vi "felhasználókl.vi"() -> ()   [LabVIEW 2015]
panel:
  in  "Tab Control":T1(tab)
  out "Array":T2(array[cluster])
  in  "Felhasználó törlése":bool
  in  "Felhasználó módosítása":bool
  in  "Felhasználó hozzáadása":bool
  in  "Felhasználó kiválasztása":string(combo)
  in  "peoples mod":T3
  in  "peoples ins":T3
  in  "Hét kiválasztása":string(combo)
  out "Waveform Chart":waveform(i32)[](graph)
  in  "Felhasználó":string
  out "Mostani hét":string
  out "Array 2":T4(array[cluster]) {"Date" format="%<%H:%M\n%Y/%m/%d>T"; "Time" format="%<%H:%M>T"}
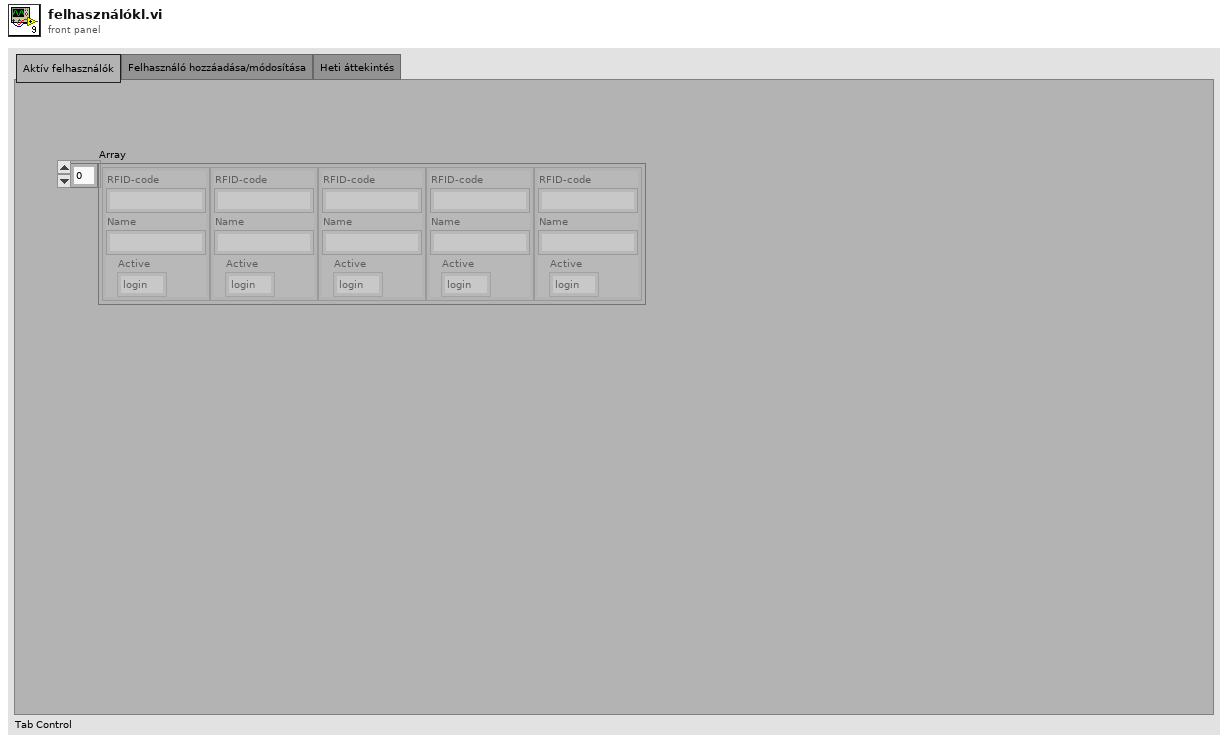
[diagram p1: front panel]
types:
  T1 = enum32{"Aktív felhasználók", "Felhasználó hozzáadása/módosítása", "Heti áttekintés"}
  T2 = cluster{"RFID-code":string, "Name":string, "Active":enum16{"login", "logout"}}[]
  T3 = cluster{"RFID-code":string, "Name":string, "Active":enum16{"login", "logout"}}
  T4 = cluster{"Name":string, "Date":timestamp, "Time":timestamp}[]
  T5 = cluster{"Name":string, "Date":timestamp, "Time":timestamp}
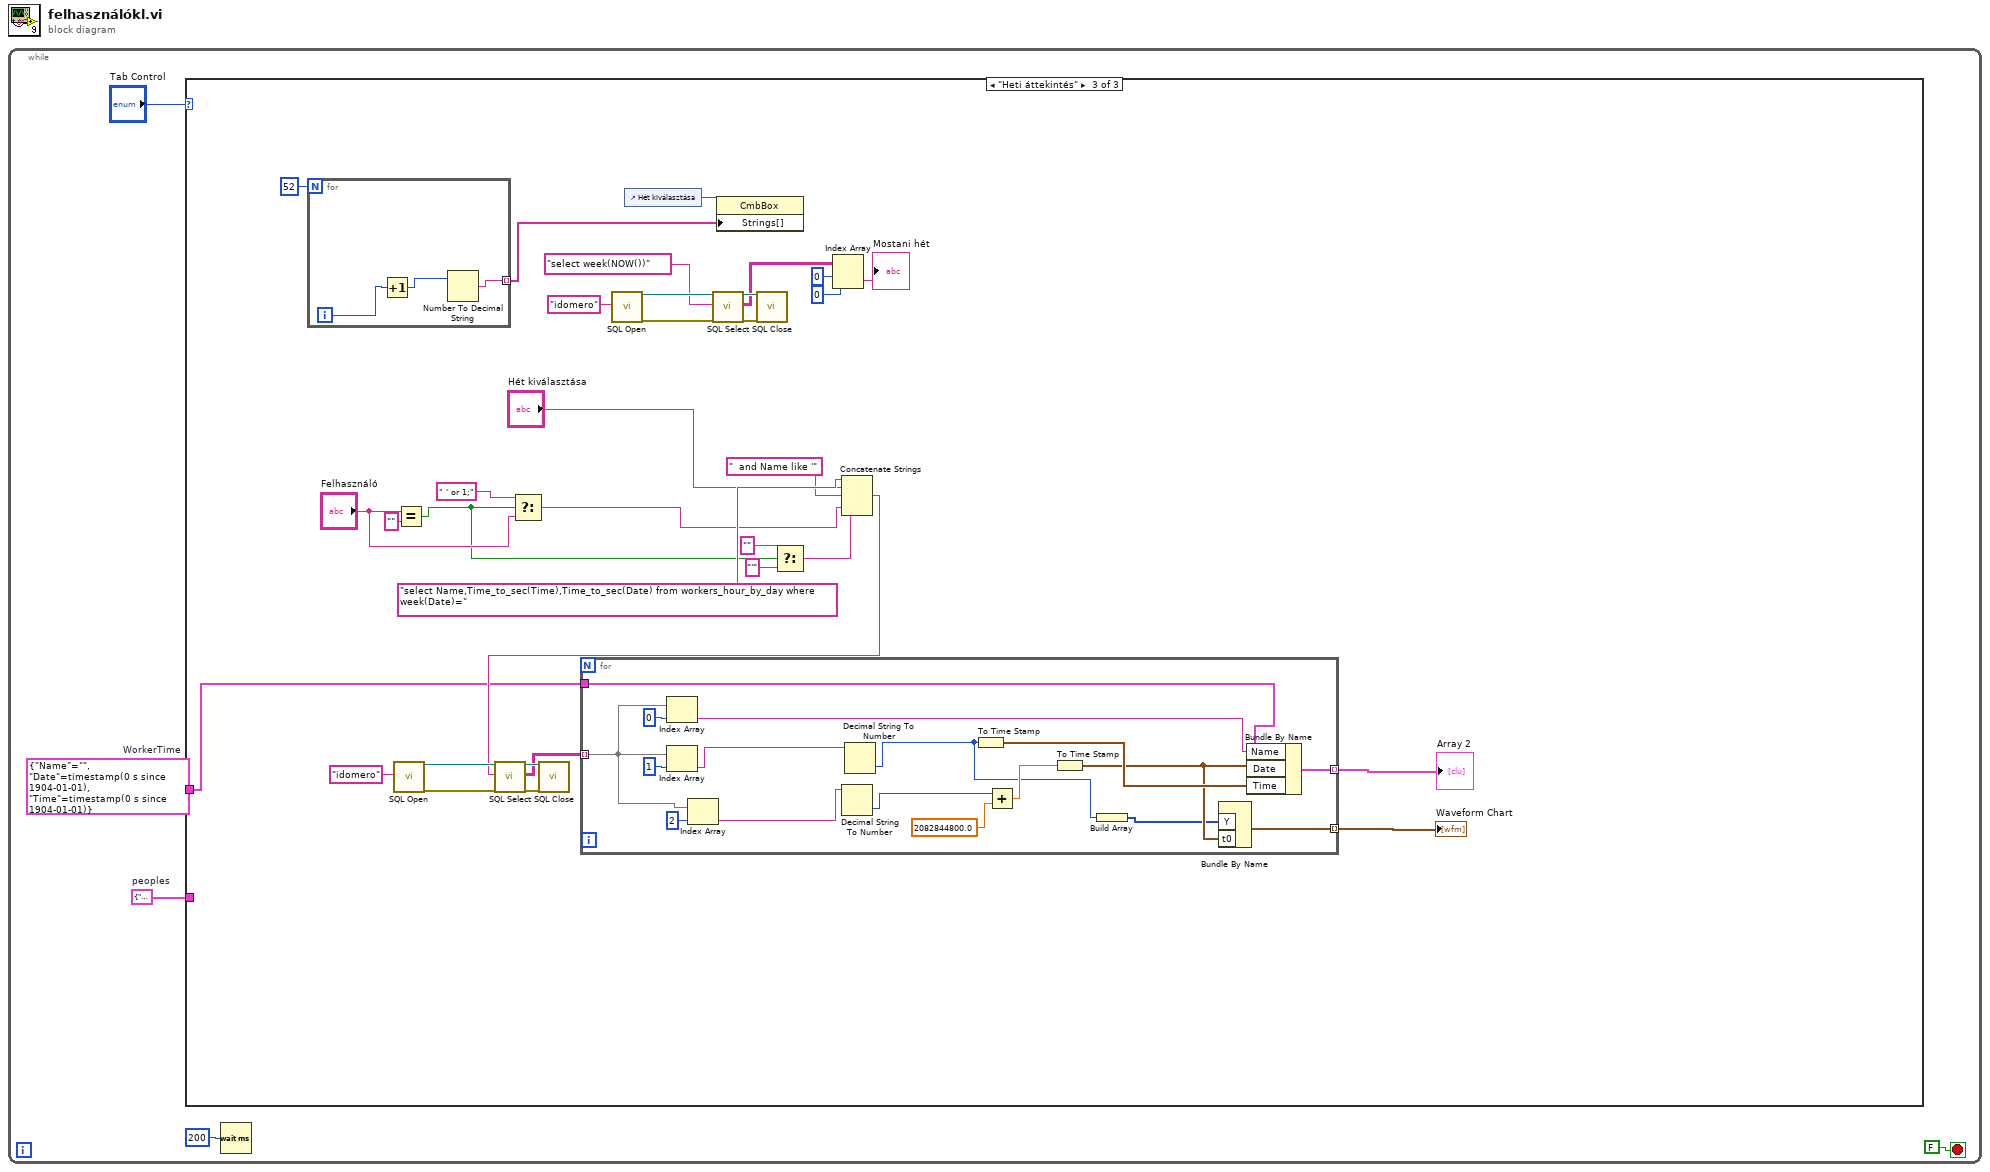
[diagram p0: block diagram]
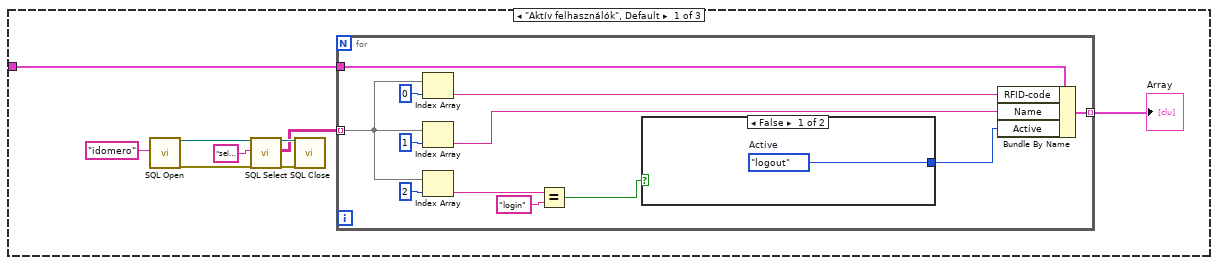
[diagram p2: hidden frame]
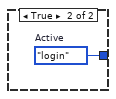
[diagram p3: hidden frame]
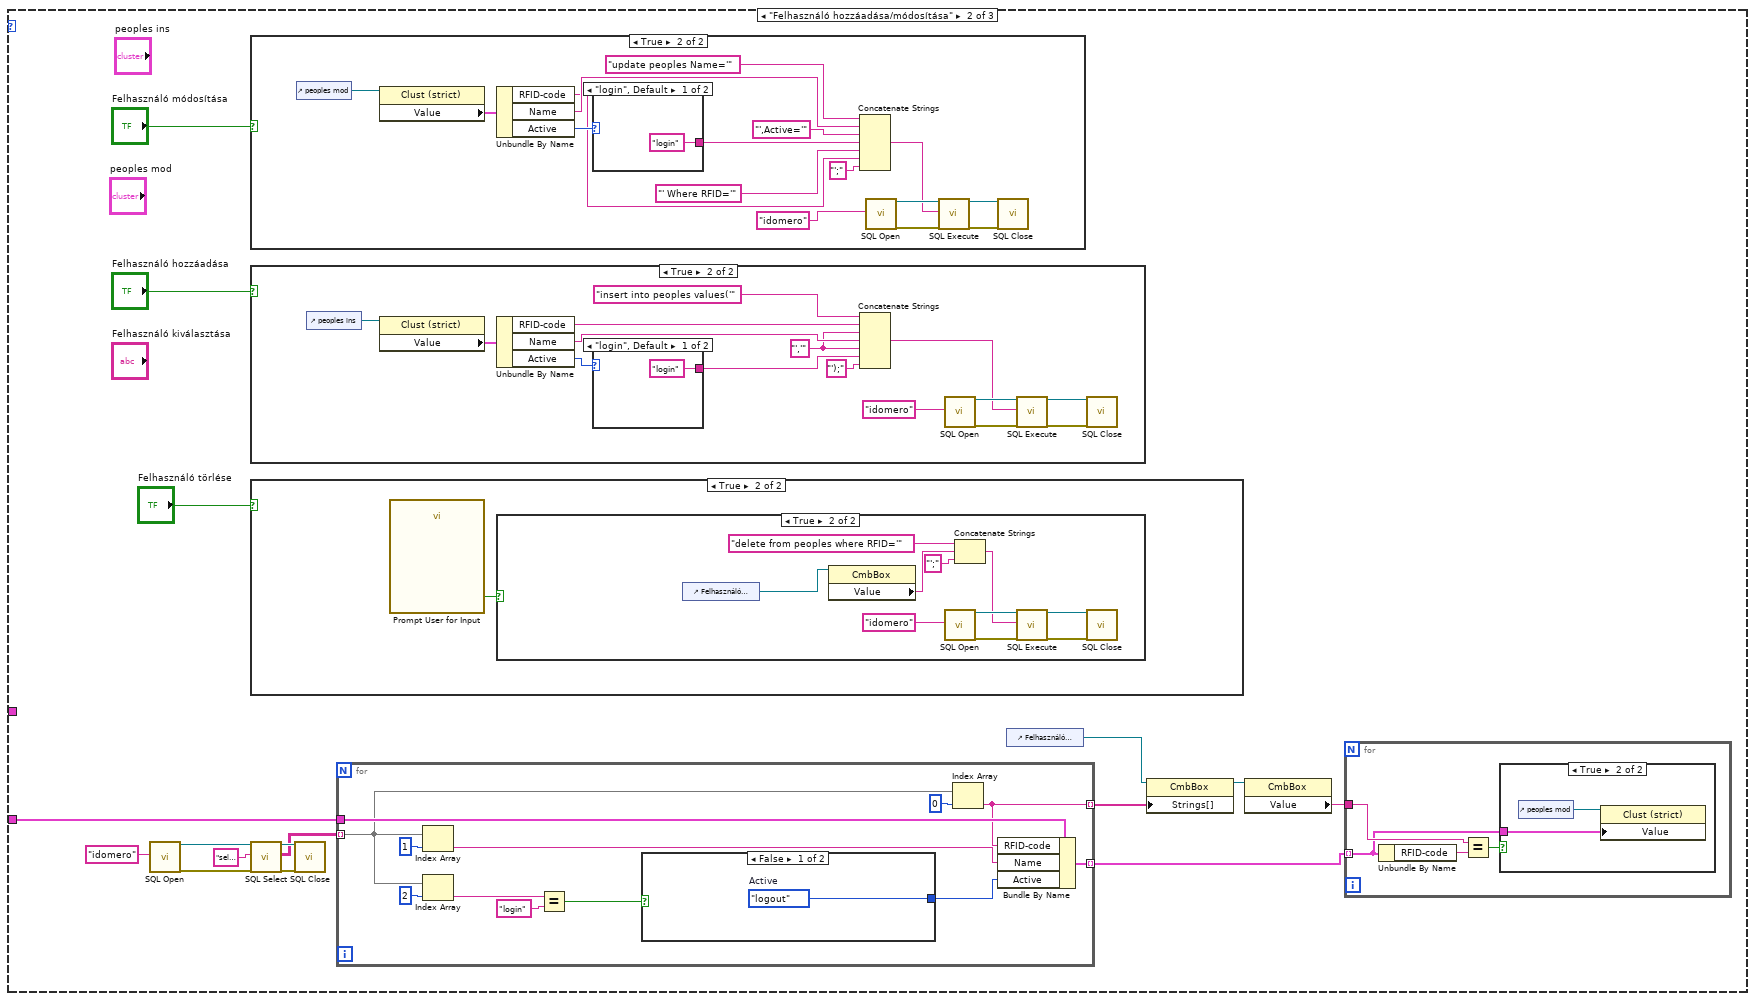
[diagram p4: hidden frame]
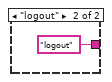
[diagram p8: hidden frame]
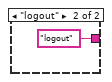
[diagram p10: hidden frame]
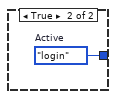
[diagram p12: hidden frame]
diagram:
  n1 = while {
    stop <- FALSE stop-if-true
    w1 = T5 {"Name"="", "Date"=timestamp(0 s since 1904-01-01), "Time"=timestamp(0 s since 1904-01-01)}  # WorkerTime
    w2 = T3 {"RFID-code"="", "Name"="", "Active"=enum."login"}  # peoples
    n2 = case shown="\"Heti áttekintés\"" "Tab Control" {
      tunnel: w2 -> [w8 w38 _]
      tunnel: w1 -> [_ _ w127]
      frame "Aktív felhasználók", Default {
        n3 = call <vilib>:"SQL Open.vi"("ConnectionString In"="idomero") -> ("Connection Out"=w13:refnum<k7>, "Error out"=w12:errorcluster)  [unwired: 17 in]
        n4 = call <vilib>:"SQL Select.vi"("Connection In"=w13, "SQL Query"="select * from peoples", "Error in (no error)"=w12) -> ("Connection Out"=w10:refnum<k7>, "Data"=w7:string[][], "Error out"=w9:errorcluster)  [unwired: 14 in]
        n5 = call <vilib>:"SQL Close.vi"("Connection In"=w10, "Error in (no error)"=w9) -> ()  [unwired: 17 in, 1 out]
        n6 = for {
          tunnel: w8 -> [w26]
          tunnel: w7 -> [w23] mode=indexing
          tunnel: [w15] -> w6 mode=indexing
          n7 = Index Array(array=w23, index=0) -> (element=w21:string)
          n8 = Index Array(array=w23, index=1) -> (element=w20:string)
          n9 = Index Array(array=w23, index=2) -> (element=w19:string)
          n10 = Equal?(x=w19, y="login") -> (x = y?=w17:bool)
          n11 = case shown="False" w17 {
            tunnel: [w27 w28] -> w16
            frame False {
              w27 = enum16{"login", "logout"}."logout"  # Active
            }
            frame True {
              w28 = enum16{"login", "logout"}."login"  # Active
            }
          }
          n12 = Bundle By Name(cluster=w26, "RFID-code"=w21, "Name"=w20, "Active"=w16) -> (w15:T3)
        }
        "Array" <- w6
      }
      frame "Felhasználó hozzáadása/módosítása" {
        n13 = call <vilib>:"SQL Open.vi"("ConnectionString In"="idomero") -> ("Connection Out"=w43:refnum<k7>, "Error out"=w42:errorcluster)  [unwired: 17 in]
        n14 = case shown="True" "Felhasználó módosítása" {
          frame False {
          }
          frame True {
            n15 = control-ref of="peoples mod"() -> (w62:refnum<vi>)
            n16 = property class="Clust (strict)"(reference=w62) -> ("Value"=w64:T3)  [unwired: 1 in, 2 out]
            n17 = Unbundle By Name(w64) -> ("RFID-code"=w57:string, "Name"=w61:string, "Active"=w63:enum16{"login", "logout"})
            n18 = case shown="\"login\", Default" w63 {
              tunnel: ["login" "logout"] -> w59
              frame "login", Default {
              }
              frame "logout" {
              }
            }
            n19 = Concatenate Strings("update peoples Name='" ("string"), w61, "',Active='" ("string"), w59, "' Where RFID='" ("string"), w57, "';" ("string")) -> (w66:string)
            n20 = call <vilib>:"SQL Open.vi"("ConnectionString In"="idomero") -> ("Connection Out"=w70:refnum<k7>, "Error out"=w69:errorcluster)  [unwired: 17 in]
            n21 = call <vilib>:"SQL Execute.vi"("Connection In"=w70, "SQL Query"=w66, "Error in (no error)"=w69) -> ("Connection Out"=w68:refnum<k7>, "Error out"=w67:errorcluster)  [unwired: 15 in]
            n22 = call <vilib>:"SQL Close.vi"("Connection In"=w68, "Error in (no error)"=w67) -> ()  [unwired: 17 in, 1 out]
          }
        }
        n23 = case shown="True" "Felhasználó hozzáadása" {
          frame False {
          }
          frame True {
            w77 = "','" ("string")
            n24 = control-ref of="peoples ins"() -> (w81:refnum<vi>)
            n25 = property class="Clust (strict)"(reference=w81) -> ("Value"=w80:T3)  [unwired: 1 in, 2 out]
            n26 = Unbundle By Name(w80) -> ("RFID-code"=w79:string, "Name"=w78:string, "Active"=w76:enum16{"login", "logout"})
            n27 = case shown="\"login\", Default" w76 {
              tunnel: ["login" "logout"] -> w75
              frame "login", Default {
              }
              frame "logout" {
              }
            }
            n28 = Concatenate Strings("insert into peoples values('" ("string"), w79, w77, w78, w77, w75, "');" ("string")) -> (w83:string)
            n29 = call <vilib>:"SQL Open.vi"("ConnectionString In"="idomero") -> ("Connection Out"=w87:refnum<k7>, "Error out"=w86:errorcluster)  [unwired: 17 in]
            n30 = call <vilib>:"SQL Execute.vi"("Connection In"=w87, "SQL Query"=w83, "Error in (no error)"=w86) -> ("Connection Out"=w85:refnum<k7>, "Error out"=w84:errorcluster)  [unwired: 15 in]
            n31 = call <vilib>:"SQL Close.vi"("Connection In"=w85, "Error in (no error)"=w84) -> ()  [unwired: 17 in, 1 out]
          }
        }
        n32 = case shown="True" "Felhasználó törlése" {
          frame False {
          }
          frame True {
            n33 = call "Prompt User for Input"() -> ("Igen"=w45:bool)  [unwired: 17 in, 2 out]
            n34 = case shown="True" w45 {
              frame False {
              }
              frame True {
                n35 = control-ref of="Felhasználó kiválasztása"() -> (w50:refnum<vi>)
                n36 = property class="CmbBox"(reference=w50) -> ("Value"=w48:string)  [unwired: 1 in, 2 out]
                n37 = call <vilib>:"SQL Open.vi"("ConnectionString In"="idomero") -> ("Connection Out"=w54:refnum<k7>, "Error out"=w53:errorcluster)  [unwired: 17 in]
                n38 = Concatenate Strings("delete from peoples where RFID='" ("string"), w48, "';" ("string")) -> (w46:string)
                n39 = call <vilib>:"SQL Execute.vi"("Connection In"=w54, "SQL Query"=w46, "Error in (no error)"=w53) -> ("Connection Out"=w52:refnum<k7>, "Error out"=w51:errorcluster)  [unwired: 15 in]
                n40 = call <vilib>:"SQL Close.vi"("Connection In"=w52, "Error in (no error)"=w51) -> ()  [unwired: 17 in, 1 out]
              }
            }
          }
        }
        n41 = call <vilib>:"SQL Select.vi"("Connection In"=w43, "SQL Query"="select * from peoples", "Error in (no error)"=w42) -> ("Connection Out"=w40:refnum<k7>, "Data"=w37:string[][], "Error out"=w39:errorcluster)  [unwired: 14 in]
        n42 = call <vilib>:"SQL Close.vi"("Connection In"=w40, "Error in (no error)"=w39) -> ()  [unwired: 17 in, 1 out]
        n43 = for {
          tunnel: w38 -> [w108]
          tunnel: w37 -> [w105] mode=indexing
          tunnel: [w98] -> w33 mode=indexing
          tunnel: [w97] -> w35 mode=indexing
          n44 = Index Array(array=w105, index=1) -> (element=w103:string)
          n45 = Index Array(array=w105, index=2) -> (element=w102:string)
          n46 = Equal?(x=w102, y="login") -> (x = y?=w100:bool)
          n47 = case shown="False" w100 {
            tunnel: [w109 w110] -> w99
            frame False {
              w109 = enum16{"login", "logout"}."logout"  # Active
            }
            frame True {
              w110 = enum16{"login", "logout"}."login"  # Active
            }
          }
          n48 = Index Array(array=w105, index=0) -> (element=w97:string)
          n49 = Bundle By Name(cluster=w108, "RFID-code"=w97, "Name"=w103, "Active"=w99) -> (w98:T3)
        }
        n50 = control-ref of="Felhasználó kiválasztása"() -> (w36:refnum<vi>)
        n51 = property class="CmbBox"(reference=w36, "Strings[]"=w35) -> (reference out=w34:refnum<vi>)  [unwired: 1 in, 1 out]
        n52 = property class="CmbBox"(reference=w34) -> ("Value"=w32:string)  [unwired: 1 in, 2 out]
        n53 = for {
          tunnel: w33 -> [w91] mode=indexing
          tunnel: w32 -> [w93]
          n54 = Unbundle By Name(w91) -> ("RFID-code"=w94:string)
          n55 = Equal?(x=w93, y=w94) -> (x = y?=w92:bool)
          n56 = case shown="True" w92 {
            tunnel: w91 -> [_ w95]
            frame False {
            }
            frame True {
              n57 = control-ref of="peoples mod"() -> (w96:refnum<vi>)
              n58 = property class="Clust (strict)"(reference=w96, "Value"=w95) -> ()  [unwired: 1 in, 2 out]
            }
          }
        }
      }
      frame "Heti áttekintés" {
        n59 = for {
          N: 52 -> [_]
          tunnel: [w145] -> w136 mode=indexing
          i -> [w147]
          n60 = Increment(x=w147) -> (x+1=w146:i32)
          n61 = Number To Decimal String(number=w146) -> (decimal integer string=w145:string)  [unwired: 1 in]
        }
        n62 = call <vilib>:"SQL Open.vi"("ConnectionString In"="idomero") -> ("Connection Out"=w143:refnum<k7>, "Error out"=w142:errorcluster)  [unwired: 17 in]
        n63 = Equal?(x="Felhasználó", y="") -> (x = y?=w125:bool)
        n64 = Select(t=" ' or 1;", s=w125, f="Felhasználó") -> (s? t:f=w128:string)
        n65 = call <vilib>:"SQL Open.vi"("ConnectionString In"="idomero") -> ("Connection Out"=w121:refnum<k7>, "Error out"=w120:errorcluster)  [unwired: 17 in]
        n66 = control-ref of="Hét kiválasztása"() -> (w137:refnum<vi>)
        n67 = call <vilib>:"SQL Select.vi"("Connection In"=w121, "SQL Query"="select week(NOW())", "Error in (no error)"=w120) -> ("Connection Out"=w119:refnum<k7>, "Data"=w116:string[][], "Error out"=w118:errorcluster)  [unwired: 14 in]
        n68 = property class="CmbBox"(reference=w137, "Strings[]"=w136) -> ()  [unwired: 1 in, 2 out]
        n69 = call <vilib>:"SQL Close.vi"("Connection In"=w119, "Error in (no error)"=w118) -> ()  [unwired: 17 in, 1 out]
        n70 = Select(t="", s=w125, f="'") -> (s? t:f=w126:string)
        n71 = Index Array(array=w116, index (row)=0, index (col)=0 ("disabled index (col)")) -> (element=→"Mostani hét":string)
        n72 = Concatenate Strings("select Name,Time_to_sec(Time),Time_to_sec(Date) from workers_hour_by_day where week(Date)=" ("SQL Query"), "Hét kiválasztása", "  and Name like '" ("string"), w128, w126) -> (w132:string)
        n73 = call <vilib>:"SQL Select.vi"("Connection In"=w143, "SQL Query"=w132, "Error in (no error)"=w142) -> ("Connection Out"=w141:refnum<k7>, "Data"=w139:string[][], "Error out"=w140:errorcluster)  [unwired: 14 in]
        n74 = call <vilib>:"SQL Close.vi"("Connection In"=w141, "Error in (no error)"=w140) -> ()  [unwired: 17 in, 1 out]
        n75 = for {
          tunnel: w139 -> [w158] mode=indexing
          tunnel: w127 -> [w161]
          tunnel: [w159] -> w112 mode=indexing
          tunnel: [w151] -> w111 mode=indexing
          n76 = Index Array(array=w158, index=0) -> (element=w160:string)
          n77 = Index Array(array=w158, index=1) -> (element=w162:string)
          n78 = Index Array(array=w158, index=2) -> (element=w155:string)
          n79 = Decimal String To Number(string=w155) -> (number=w156:i32)  [unwired: 2 in, 1 out]
          n80 = Decimal String To Number(string=w162) -> (number=w148:i32)  [unwired: 2 in, 1 out]
          n81 = To Time Stamp(1:w148) -> (0:w153:timestamp)
          n82 = Add(x=w156, y=2082844800.0) -> (x+y=w150:dbl)
          n83 = To Time Stamp(1:w150) -> (0:w152:timestamp)
          n84 = Build Array(w148) -> (w149:i32[])
          n85 = Bundle By Name("Y"=w149, "t0"=w152) -> (w151:waveform(i32))  [unwired: 1 in]
          n86 = Bundle By Name(cluster=w161, "Name"=w160, "Date"=w152, "Time"=w153) -> (w159:T5)
        }
        "Waveform Chart" <- w111
        "Array 2" <- w112
      }
    }
    n87 = Wait (ms)(milliseconds to wait=u32 200) -> ()  [unwired: 1 out]
  }
